vi "FA Data Type List.vi"(0 "FA Data And Events":T1) -> (1 "Data Type List":string[](array[string]), 2 "Tip String":string, 3 "error out":errorcluster)   [LabVIEW 2016, in "M1M3SupportEUI_Views.lvlib"]
uses:
  M1M3SupportEUI_Views.lvlib
  Typedefs/FA Data And Events.ctl
  SALLV_m1m3/DataTypes/ForceActuatorData.ctl
  SALLV_m1m3/DataTypes/logevent_ForceActuatorForceWarning.ctl
  SALLV_m1m3/DataTypes/logevent_ForceActuatorInfo.ctl
  SALLV_m1m3/DataTypes/logevent_ForceActuatorState.ctl
  SALLV_m1m3/DataTypes/logevent_ForceActuatorWarning.ctl
  SALLV_m1m3/DataTypes/logevent_AppliedAberrationForces.ctl
  SALLV_m1m3/DataTypes/logevent_AppliedAccelerationForces.ctl
  SALLV_m1m3/DataTypes/logevent_AppliedActiveOpticForces.ctl
  SALLV_m1m3/DataTypes/logevent_AppliedAzimuthForces.ctl
  SALLV_m1m3/DataTypes/logevent_AppliedBalanceForces.ctl
  SALLV_m1m3/DataTypes/logevent_AppliedCylinderForces.ctl
  SALLV_m1m3/DataTypes/logevent_AppliedElevationForces.ctl
  SALLV_m1m3/DataTypes/logevent_AppliedForces.ctl
  SALLV_m1m3/DataTypes/logevent_AppliedOffsetForces.ctl
  SALLV_m1m3/DataTypes/logevent_AppliedStaticForces.ctl
  SALLV_m1m3/DataTypes/logevent_AppliedThermalForces.ctl
  SALLV_m1m3/DataTypes/logevent_AppliedVelocityForces.ctl
  SALLV_m1m3/DataTypes/logevent_RejectedAberrationForces.ctl
  SALLV_m1m3/DataTypes/logevent_RejectedAccelerationForces.ctl
  SALLV_m1m3/DataTypes/logevent_RejectedActiveOpticForces.ctl
  SALLV_m1m3/DataTypes/logevent_RejectedAzimuthForces.ctl
  SALLV_m1m3/DataTypes/logevent_RejectedBalanceForces.ctl
  SALLV_m1m3/DataTypes/logevent_RejectedCylinderForces.ctl
  SALLV_m1m3/DataTypes/logevent_RejectedElevationForces.ctl
  SALLV_m1m3/DataTypes/logevent_RejectedForces.ctl
  SALLV_m1m3/DataTypes/logevent_RejectedOffsetForces.ctl
  SALLV_m1m3/DataTypes/logevent_RejectedStaticForces.ctl
  SALLV_m1m3/DataTypes/logevent_RejectedThermalForces.ctl
  SALLV_m1m3/DataTypes/logevent_RejectedVelocityForces.ctl
  SALLV_m1m3/SALLV_m1m3.lvlib
  Typedefs/M1M3SupportEUI_TypeDefs.lvlib
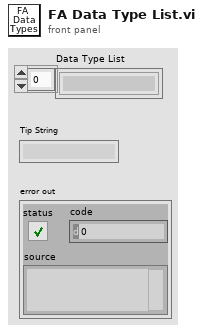
[diagram p1: front panel]
types:
  T1 = typedef "M1M3SupportEUI_TypeDefs.lvlib/FA Data And Events.ctl" = cluster{"ForceActuatorData":T2, "logevent_ForceActuatorForceWarning":T3, "logevent_ForceActuatorInfo":T4, "logevent_ForceActuatorState":T5, "logevent_ForceActuatorWarning":T6, "logevent_AppliedAberrationForces":T7, "logevent_AppliedAccelerationForces":T8, "logevent_AppliedActiveOpticForces":T9, "logevent_AppliedAzimuthForces":T10, "logevent_AppliedBalanceForces":T11, "logevent_AppliedCylinderForces":T12, "logevent_AppliedElevationForces":T13, "logevent_AppliedForces":T14, "logevent_AppliedOffsetForces":T15, "logevent_AppliedStaticForces":T16, "logevent_AppliedThermalForces":T17, "logevent_AppliedVelocityForces":T18, "logevent_RejectedAberrationForces":T19, "logevent_RejectedAccelerationForces":T20, "logevent_RejectedActiveOpticForces":T21, "logevent_RejectedAzimuthForces":T22, "logevent_RejectedBalanceForces":T23, "logevent_RejectedCylinderForces":T24, "logevent_RejectedElevationForces":T25, "logevent_RejectedForces":T26, "logevent_RejectedOffsetForces":T27, "logevent_RejectedStaticForces":T28, "logevent_RejectedThermalForces":T29, "logevent_RejectedVelocityForces":T30}
  T2 = typedef "SALLV_m1m3.lvlib/ForceActuatorData.ctl" = cluster{"Timestamp":dbl, "PrimaryCylinderForce[156]":sgl[], "SecondaryCylinderForce[112]":sgl[], "XForce[12]":sgl[], "YForce[100]":sgl[], "ZForce[156]":sgl[], "Fx":sgl, "Fy":sgl, "Fz":sgl, "Mx":sgl, "My":sgl, "Mz":sgl, "ForceMagnitude":sgl}
  T3 = typedef "SALLV_m1m3.lvlib/logevent_ForceActuatorForceWarning.ctl" = cluster{"Timestamp":dbl, "AnyWarning":bool, "AnyPrimaryAxisMeasuredForceWarning":bool, "PrimaryAxisMeasuredForceWarning[156]":bool[], "AnySecondaryAxisMeasuredForceWarning":bool, "SecondaryAxisMeasuredForceWarning[156]":bool[], "AnyPrimaryAxisFollowingErrorWarning":bool, "PrimaryAxisFollowingErrorWarning[156]":bool[], "AnySecondaryAxisFollowingErrorWarning":bool, "SecondaryAxisFollowingErrorWarning[156]":bool[], "priority":i32}
  T4 = typedef "SALLV_m1m3.lvlib/logevent_ForceActuatorInfo.ctl" = cluster{"Timestamp":dbl, "ReferenceId[156]":i16[], "XDataReferenceId[12]":i16[], "YDataReferenceId[100]":i16[], "ZDataReferenceId[156]":i16[], "ActuatorType[156]":i16[], "ActuatorOrientation[156]":i16[], "ModbusSubnet[156]":i16[], "ModbusAddress[156]":i16[], "XPosition[156]":sgl[], "YPosition[156]":sgl[], "ZPosition[156]":sgl[], "ILCUniqueId[156]":i64[], "ILCApplicationType[156]":i16[], "NetworkNodeType[156]":i16[], "ILCSelectedOptions[156]":i16[], "NetworkNodeOptions[156]":i16[], "MajorRevision[156]":i16[], "MinorRevision[156]":i16[], "ADCScanRate[156]":i16[], "MainPrimaryCylinderCoefficient[156]":sgl[], "MainSecondaryCylinderCoefficient[156]":sgl[], "MainPrimaryCylinderLoadCellOffset[156]":sgl[], "MainSecondaryCylinderLoadCellOffset[156]":sgl[], "MainPrimaryCylinderLoadCellSensitivity[156]":sgl[], "MainSecondaryCylinderLoadCellSensitivity[156]":sgl[], "BackupPrimaryCylinderCoefficient[156]":sgl[], "BackupSecondaryCylinderCoefficient[156]":sgl[], "BackupPrimaryCylinderLoadCellOffset[156]":sgl[], "BackupSecondaryCylinderLoadCellOffset[156]":sgl[], "BackupPrimaryCylinderLoadCellSensitivity[156]":sgl[], "BackupSecondaryCylinderLoadCellSensitivity[156]":sgl[], "MezzaninePrimaryCylinderGain[156]":sgl[], "MezzanineSecondaryCylinderGain[156]":sgl[], "MezzanineUniqueId[156]":i64[], "MezzanineFirmwareType[156]":i16[], "MezzanineMajorRevision[156]":i16[], "MezzanineMinorRevision[156]":i16[], "priority":i32}
  T5 = typedef "SALLV_m1m3.lvlib/logevent_ForceActuatorState.ctl" = cluster{"Timestamp":dbl, "ILCState[156]":i16[], "SlewFlag":bool, "StaticForcesApplied":bool, "ElevationForcesApplied":bool, "AzimuthForcesApplied":bool, "ThermalForcesApplied":bool, "OffsetForcesApplied":bool, "AccelerationForcesApplied":bool, "VelocityForcesApplied":bool, "ActiveOpticForcesApplied":bool, "AberrationForcesApplied":bool, "BalanceForcesApplied":bool, "SupportPercentage":sgl, "priority":i32}
  T6 = typedef "SALLV_m1m3.lvlib/logevent_ForceActuatorWarning.ctl" = cluster{"Timestamp":dbl, "AnyWarning":bool, "AnyMajorFault":bool, "MajorFault[156]":bool[], "AnyMinorFault":bool, "MinorFault[156]":bool[], "AnyFaultOverride":bool, "FaultOverride[156]":bool[], "AnyMainCalibrationError":bool, "MainCalibrationError[156]":bool[], "AnyBackupCalibrationError":bool, "BackupCalibrationError[156]":bool[], "AnyMezzanineError":bool, "MezzanineError[156]":bool[], "AnyMezzanineBootloaderActive":bool, "MezzanineBootloaderActive[156]":bool[], "AnyUniqueIdCRCError":bool, "UniqueIdCRCError[156]":bool[], "AnyApplicationTypeMismatch":bool, "ApplicationTypeMismatch[156]":bool[], "AnyApplicationMissing":bool, "ApplicationMissing[156]":bool[], "AnyApplicationCRCMismatch":bool, "ApplicationCRCMismatch[156]":bool[], "AnyOneWireMissing":bool, "OneWireMissing[156]":bool[], "AnyOneWire1Mismatch":bool, "OneWire1Mismatch[156]":bool[], "AnyOneWire2Mismatch":bool, "OneWire2Mismatch[156]":bool[], "AnyWatchdogReset":bool, "WatchdogReset[156]":bool[], "AnyBrownOut":bool, "BrownOut[156]":bool[], "AnyEventTrapReset":bool, "EventTrapReset[156]":bool[], "AnySSRPowerFault":bool, "SSRPowerFault[156]":bool[], "AnyAuxPowerFault":bool, "AuxPowerFault[156]":bool[], "AnyMezzaninePowerFault":bool, "MezzaninePowerFault[156]":bool[], "AnyMezzanineCurrentAmp1Fault":bool, "MezzanineCurrentAmp1Fault[156]":bool[], "AnyMezzanineCurrentAmp2Fault":bool, "MezzanineCurrentAmp2Fault[156]":bool[], "AnyMezzanineUniqueIdCRCError":bool, "MezzanineUniqueIdCRCError[156]":bool[], "AnyMezzanineMainCalibrationError":bool, "MezzanineMainCalibrationError[156]":bool[], "AnyMezzanineBackupCalibrationError":bool, "MezzanineBackupCalibrationError[156]":bool[], "AnyMezzanineEventTrapReset":bool, "MezzanineEventTrapReset[156]":bool[], "AnyMezzanineApplicationMissing":bool, "MezzanineApplicationMissing[156]":bool[], "AnyMezzanineApplicationCRCMismatch":bool, "MezzanineApplicationCRCMismatch[156]":bool[], "AnyILCFault":bool, "ILCFault[156]":bool[], "AnyBroadcastCounterWarning":bool, "BroadcastCounterWarning[156]":bool[], "priority":i32}
  T7 = typedef "SALLV_m1m3.lvlib/logevent_AppliedAberrationForces.ctl" = cluster{"Timestamp":dbl, "ZForces[156]":sgl[], "Fz":sgl, "Mx":sgl, "My":sgl, "priority":i32}
  T8 = typedef "SALLV_m1m3.lvlib/logevent_AppliedAccelerationForces.ctl" = cluster{"Timestamp":dbl, "XForces[12]":sgl[], "YForces[100]":sgl[], "ZForces[156]":sgl[], "Fx":sgl, "Fy":sgl, "Fz":sgl, "Mx":sgl, "My":sgl, "Mz":sgl, "ForceMagnitude":sgl, "priority":i32}
  T9 = typedef "SALLV_m1m3.lvlib/logevent_AppliedActiveOpticForces.ctl" = cluster{"Timestamp":dbl, "ZForces[156]":sgl[], "Fz":sgl, "Mx":sgl, "My":sgl, "priority":i32}
  T10 = typedef "SALLV_m1m3.lvlib/logevent_AppliedAzimuthForces.ctl" = cluster{"Timestamp":dbl, "XForces[12]":sgl[], "YForces[100]":sgl[], "ZForces[156]":sgl[], "Fx":sgl, "Fy":sgl, "Fz":sgl, "Mx":sgl, "My":sgl, "Mz":sgl, "ForceMagnitude":sgl, "priority":i32}
  T11 = typedef "SALLV_m1m3.lvlib/logevent_AppliedBalanceForces.ctl" = cluster{"Timestamp":dbl, "XForces[12]":sgl[], "YForces[100]":sgl[], "ZForces[156]":sgl[], "Fx":sgl, "Fy":sgl, "Fz":sgl, "Mx":sgl, "My":sgl, "Mz":sgl, "ForceMagnitude":sgl, "priority":i32}
  T12 = typedef "SALLV_m1m3.lvlib/logevent_AppliedCylinderForces.ctl" = cluster{"Timestamp":dbl, "SecondaryCylinderForces[112]":i32[], "PrimaryCylinderForces[156]":i32[], "priority":i32}
  T13 = typedef "SALLV_m1m3.lvlib/logevent_AppliedElevationForces.ctl" = cluster{"Timestamp":dbl, "XForces[12]":sgl[], "YForces[100]":sgl[], "ZForces[156]":sgl[], "Fx":sgl, "Fy":sgl, "Fz":sgl, "Mx":sgl, "My":sgl, "Mz":sgl, "ForceMagnitude":sgl, "priority":i32}
  T14 = typedef "SALLV_m1m3.lvlib/logevent_AppliedForces.ctl" = cluster{"Timestamp":dbl, "XForces[12]":sgl[], "YForces[100]":sgl[], "ZForces[156]":sgl[], "Fx":sgl, "Fy":sgl, "Fz":sgl, "Mx":sgl, "My":sgl, "Mz":sgl, "ForceMagnitude":sgl, "priority":i32}
  T15 = typedef "SALLV_m1m3.lvlib/logevent_AppliedOffsetForces.ctl" = cluster{"Timestamp":dbl, "XForces[12]":sgl[], "YForces[100]":sgl[], "ZForces[156]":sgl[], "Fx":sgl, "Fy":sgl, "Fz":sgl, "Mx":sgl, "My":sgl, "Mz":sgl, "ForceMagnitude":sgl, "priority":i32}
  T16 = typedef "SALLV_m1m3.lvlib/logevent_AppliedStaticForces.ctl" = cluster{"Timestamp":dbl, "XForces[12]":sgl[], "YForces[100]":sgl[], "ZForces[156]":sgl[], "Fx":sgl, "Fy":sgl, "Fz":sgl, "Mx":sgl, "My":sgl, "Mz":sgl, "ForceMagnitude":sgl, "priority":i32}
  T17 = typedef "SALLV_m1m3.lvlib/logevent_AppliedThermalForces.ctl" = cluster{"Timestamp":dbl, "XForces[12]":sgl[], "YForces[100]":sgl[], "ZForces[156]":sgl[], "Fx":sgl, "Fy":sgl, "Fz":sgl, "Mx":sgl, "My":sgl, "Mz":sgl, "ForceMagnitude":sgl, "priority":i32}
  T18 = typedef "SALLV_m1m3.lvlib/logevent_AppliedVelocityForces.ctl" = cluster{"Timestamp":dbl, "XForces[12]":sgl[], "YForces[100]":sgl[], "ZForces[156]":sgl[], "Fx":sgl, "Fy":sgl, "Fz":sgl, "Mx":sgl, "My":sgl, "Mz":sgl, "ForceMagnitude":sgl, "priority":i32}
  T19 = typedef "SALLV_m1m3.lvlib/logevent_RejectedAberrationForces.ctl" = cluster{"Timestamp":dbl, "ZForces[156]":sgl[], "Fz":sgl, "Mx":sgl, "My":sgl, "priority":i32}
  T20 = typedef "SALLV_m1m3.lvlib/logevent_RejectedAccelerationForces.ctl" = cluster{"Timestamp":dbl, "XForces[12]":sgl[], "YForces[100]":sgl[], "ZForces[156]":sgl[], "Fx":sgl, "Fy":sgl, "Fz":sgl, "Mx":sgl, "My":sgl, "Mz":sgl, "ForceMagnitude":sgl, "priority":i32}
  T21 = typedef "SALLV_m1m3.lvlib/logevent_RejectedActiveOpticForces.ctl" = cluster{"Timestamp":dbl, "ZForces[156]":sgl[], "Fz":sgl, "Mx":sgl, "My":sgl, "priority":i32}
  T22 = typedef "SALLV_m1m3.lvlib/logevent_RejectedAzimuthForces.ctl" = cluster{"Timestamp":dbl, "XForces[12]":sgl[], "YForces[100]":sgl[], "ZForces[156]":sgl[], "Fx":sgl, "Fy":sgl, "Fz":sgl, "Mx":sgl, "My":sgl, "Mz":sgl, "ForceMagnitude":sgl, "priority":i32}
  T23 = typedef "SALLV_m1m3.lvlib/logevent_RejectedBalanceForces.ctl" = cluster{"Timestamp":dbl, "XForces[12]":sgl[], "YForces[100]":sgl[], "ZForces[156]":sgl[], "Fx":sgl, "Fy":sgl, "Fz":sgl, "Mx":sgl, "My":sgl, "Mz":sgl, "ForceMagnitude":sgl, "priority":i32}
  T24 = typedef "SALLV_m1m3.lvlib/logevent_RejectedCylinderForces.ctl" = cluster{"Timestamp":dbl, "SecondaryCylinderForces[112]":i32[], "PrimaryCylinderForces[156]":i32[], "priority":i32}
  T25 = typedef "SALLV_m1m3.lvlib/logevent_RejectedElevationForces.ctl" = cluster{"Timestamp":dbl, "XForces[12]":sgl[], "YForces[100]":sgl[], "ZForces[156]":sgl[], "Fx":sgl, "Fy":sgl, "Fz":sgl, "Mx":sgl, "My":sgl, "Mz":sgl, "ForceMagnitude":sgl, "priority":i32}
  T26 = typedef "SALLV_m1m3.lvlib/logevent_RejectedForces.ctl" = cluster{"Timestamp":dbl, "XForces[12]":sgl[], "YForces[100]":sgl[], "ZForces[156]":sgl[], "Fx":sgl, "Fy":sgl, "Fz":sgl, "Mx":sgl, "My":sgl, "Mz":sgl, "ForceMagnitude":sgl, "priority":i32}
  T27 = typedef "SALLV_m1m3.lvlib/logevent_RejectedOffsetForces.ctl" = cluster{"Timestamp":dbl, "XForces[12]":sgl[], "YForces[100]":sgl[], "ZForces[156]":sgl[], "Fx":sgl, "Fy":sgl, "Fz":sgl, "Mx":sgl, "My":sgl, "Mz":sgl, "ForceMagnitude":sgl, "priority":i32}
  T28 = typedef "SALLV_m1m3.lvlib/logevent_RejectedStaticForces.ctl" = cluster{"Timestamp":dbl, "XForces[12]":sgl[], "YForces[100]":sgl[], "ZForces[156]":sgl[], "Fx":sgl, "Fy":sgl, "Fz":sgl, "Mx":sgl, "My":sgl, "Mz":sgl, "ForceMagnitude":sgl, "priority":i32}
  T29 = typedef "SALLV_m1m3.lvlib/logevent_RejectedThermalForces.ctl" = cluster{"Timestamp":dbl, "XForces[12]":sgl[], "YForces[100]":sgl[], "ZForces[156]":sgl[], "Fx":sgl, "Fy":sgl, "Fz":sgl, "Mx":sgl, "My":sgl, "Mz":sgl, "ForceMagnitude":sgl, "priority":i32}
  T30 = typedef "SALLV_m1m3.lvlib/logevent_RejectedVelocityForces.ctl" = cluster{"Timestamp":dbl, "XForces[12]":sgl[], "YForces[100]":sgl[], "ZForces[156]":sgl[], "Fx":sgl, "Fy":sgl, "Fz":sgl, "Mx":sgl, "My":sgl, "Mz":sgl, "ForceMagnitude":sgl, "priority":i32}
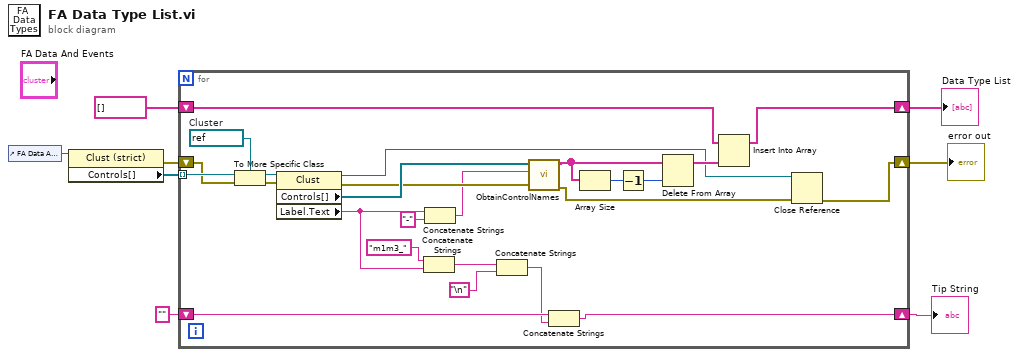
[diagram p0: block diagram]
diagram:
  n1 = control-ref of="FA Data And Events"() -> (w8:refnum<vi>)
  n2 = property class="Clust (strict)"(reference=w8) -> (error out=w6:errorcluster, "Controls[]"=w7:refnum<vi>[])  [unwired: 1 in, 1 out]
  n3 = for {
    tunnel: w7 -> [w27] mode=indexing
    shift-right: [w13] -> w3
    shift-left: w6 -> [w26]
    shift-right: [w19] -> w5
    shift-left: "" -> [w18]
    shift-right: [w16] -> w4
    shift-left: string[] [] -> [w15]
    w24 = refnum<vi> refnum  # Cluster
    n4 = To More Specific Class(target class=w24, reference=w27, error in=w26) -> (specific class reference=w25:refnum<vi>, error out=w28:errorcluster)
    n5 = property class="Clust"(reference=w25, error in=w28) -> (reference out=w12:refnum<vi>, error out=w29:errorcluster, "Controls[]"=w30:refnum<vi>[], "Label.Text"=w11:string)
    n6 = Concatenate Strings("m1m3_", w11) -> (w21:string)
    n7 = Concatenate Strings(w11, "-" ("string")) -> (w10:string)
    n8 = Concatenate Strings(w21, "\n") -> (w17:string)
    n9 = call "ObtainControlNames.vi"("error in (no error)"=w29, "AddedPrefix"=w10, "ControlRefnumArray"=w30) -> ("error out"=w14:errorcluster, "ControlNamesArray"=w23:string[])  [unwired: 7 in]
    n10 = Concatenate Strings(w18, w17) -> (w19:string)
    n11 = Array Size(array=w23) -> (size(s)=w31:i32)
    n12 = Decrement(x=w31) -> (x-1=w32:i32)
    n13 = Delete From Array(array=w23, index=w32) -> (array with subset deleted=w33:string[])  [unwired: 1 in, 1 out]
    n14 = Insert Into Array(array=w15, new element=w33) -> (w16:string[])  [unwired: 1 in]
    n15 = Close Reference(reference=w12, error in (no error)=w14) -> (error out=w13:errorcluster)
  }
  "Data Type List" <- w4
  "Tip String" <- w5
  "error out" <- w3
